vi "Conditionally Append String to Array.vi"(9 "배열에 추가할 텍스트":string, 10 "추가?":bool, 11 "문자열 배열 입력":string[](array[string])) -> (3 "문자열 배열 출력":string[](array[string]))   [LabVIEW 2010]
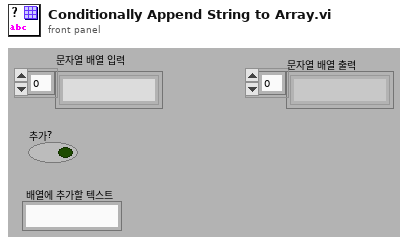
[diagram p1: front panel]
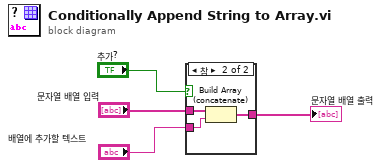
[diagram p0: block diagram]
diagram:
  n1 = case shown="참" "추가?" {
    tunnel: "배열에 추가할 텍스트" -> [_ w7]
    tunnel: "문자열 배열 입력" -> [w5 w8]
    tunnel: [w5 w6] -> w1
    frame False {
    }
    frame True {
      n2 = Build Array (concatenate)(w8, w7) -> (w6:string[])
    }
  }
  "문자열 배열 출력" <- w1
